vi "Write AO task.vi"(8 "error in (no error)":errorcluster, 10 "AO task":refnum<k21>, 11 "DAQmx Lockin Digitizer Driver in":refnum<class "DAQmx Lockin Digitizer Driver.lvclass">) -> (0 "error out":errorcluster, 3 "DAQmx Lockin Digitizer Driver out":refnum<class "DAQmx Lockin Digitizer Driver.lvclass">)   [LabVIEW 2021, in "DAQmx Lockin Digitizer Driver.lvclass"]
uses:
  DAQmx Lockin Digitizer Driver.lvclass
  DAQmx Lockin Digitizer Driver.lvclass/DAQmx Lockin Digitizer Driver.ctl
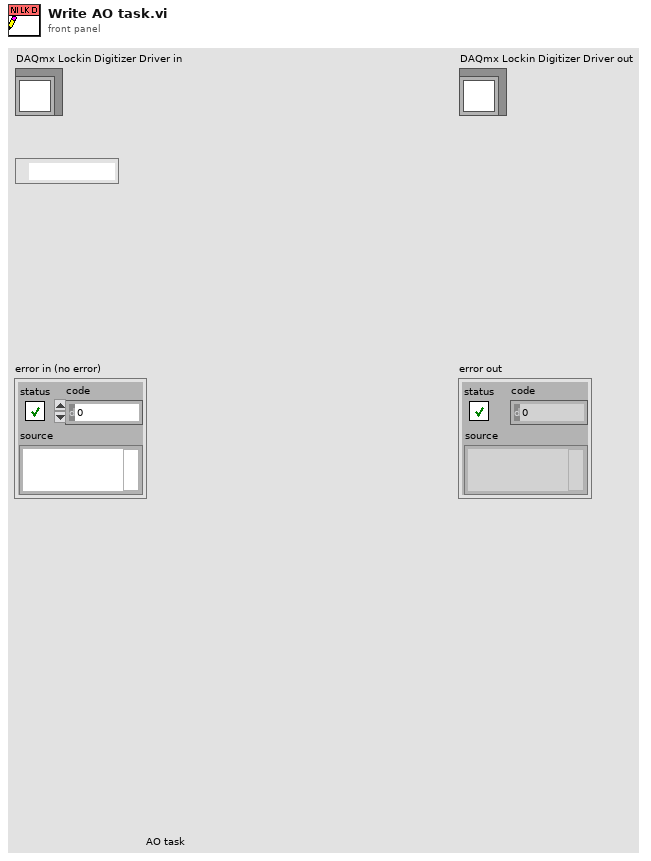
[diagram p1: front panel]
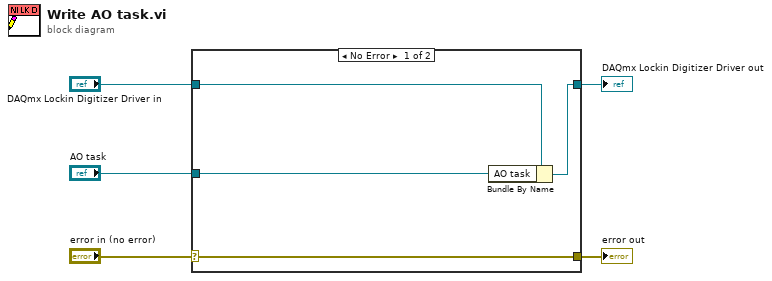
[diagram p0: block diagram]
diagram:
  n1 = case shown="No Error" "error in (no error)" {
    selector: "error in (no error)" -> [w9 w10]
    tunnel: [w9 w10] -> w4
    tunnel: [w7 w11] -> w2
    tunnel: "DAQmx Lockin Digitizer Driver in" -> [w8 w11]
    tunnel: "AO task" -> [w6 _]
    frame No Error {
      n2 = Bundle By Name(cluster=w8, "AO task"=w6) -> (w7:refnum<class "DAQmx Lockin Digitizer Driver.lvclass">)
    }
    frame Error {
    }
  }
  "error out" <- w4
  "DAQmx Lockin Digitizer Driver out" <- w2
